vi "VRM.Ramp to Set.vi"(6 "Axis":T1=enum."Z", 8 "error in (no error)":errorcluster, 11 "Instrument.VRM in":refnum<class "Instrument.OxfordVRM.lvclass">) -> (0 "error out":errorcluster, 2 "Response":string[](array[string]), 3 "Instrument.VRM out":refnum<class "Instrument.OxfordVRM.lvclass">)   [LabVIEW 2019, in "Instrument.OxfordVRM.lvclass"]
uses:
  Instrument.OxfordVRM.lvclass
  Typedefs/VRM Magnet Axis--Enum.ctl
  <instrlib>/Mercury iXX/Public/Libraries/Magnet/Controls/PSU Actions.ctl
  <instrlib>/Mercury iXX/Public/Libraries/Magnet.lvlib
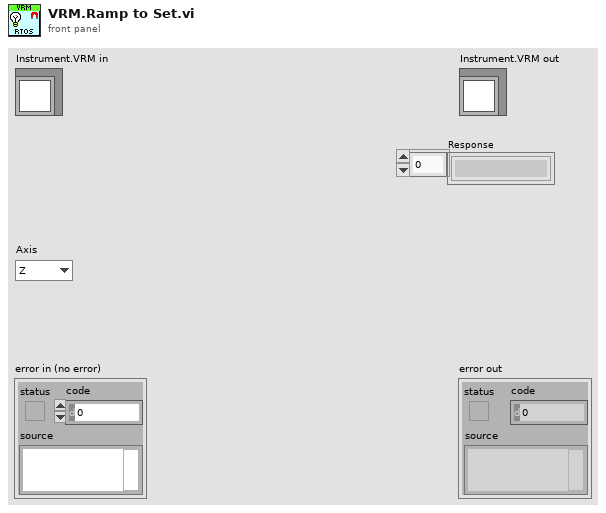
[diagram p1: front panel]
types:
  T1 = typedef "Instrument.OxfordVRM.lvclass/VRM Magnet Axis--Enum.ctl" = enum16{"X", "Y", "Z", "ALL"}
  T2 = typedef "Mercury iXX.lvlib/Magnet.lvlib/PSU Actions.ctl" = string
  T3 = typedef "Instrument.Cryostat.lvclass/Magnet Axis--Enum.ctl" = enum16{"X", "Y", "Z"}
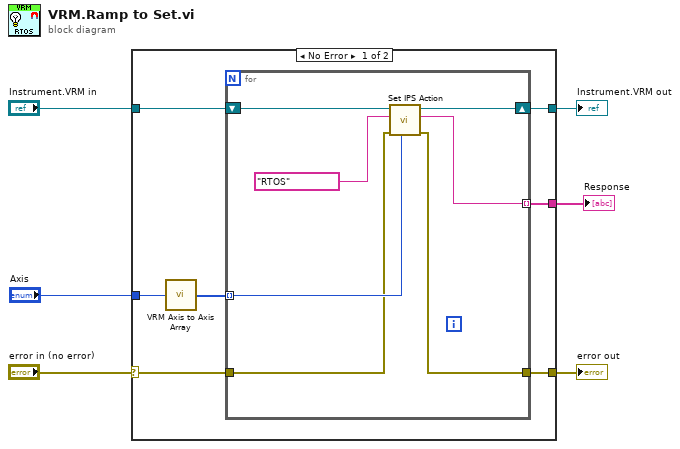
[diagram p0: block diagram]
diagram:
  n1 = case shown="No Error" "error in (no error)" {
    selector: "error in (no error)" -> [w12 w22]
    tunnel: [w11 w22] -> w5
    tunnel: [w10 w21] -> w3
    tunnel: "Instrument.VRM in" -> [w13 w21]
    tunnel: "Axis" -> [w9 _]
    tunnel: [w7 _] -> w1
    frame No Error {
      n2 = call "VRM Axis to Axis Array.vi"("Axis"=w9) -> ("Axis Array"=w8:T3[])
      n3 = for {
        shift-right: [w19] -> w10
        shift-left: w13 -> [w17]
        tunnel: w8 -> [w20] mode=indexing
        tunnel: w12 -> [w16]
        tunnel: [w18] -> w11
        tunnel: [w14] -> w7 mode=indexing
        n4 = call "Set IPS Action.vi"("Axis"=w20, "error in (no error)"=w16, "PSU Act Stat"=T2 "RTOS", "Instrument.OxfordVRM in"=w17) -> ("error out"=w18:errorcluster, "Response"=w14:string, "Instrument.OxfordVRM out"=w19:refnum<class "Instrument.OxfordVRM.lvclass">)  [unwired: 5 in]
      }
    }
    frame Error {
    }
  }
  "error out" <- w5
  "Instrument.VRM out" <- w3
  "Response" <- w1
